vi "IDByteDecoder.vi"(0 "byte1":string="Ò") -> (1 "Type de donnee (ID)":i32, 2 "Ordre/ /(info)":bool, 3 "marche normale/ /(debug)":bool)   [LabVIEW 2010]
doc: "Décodage d'un octet de type de données"
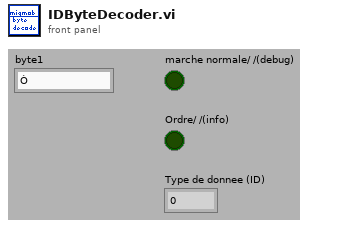
[diagram p1: front panel]
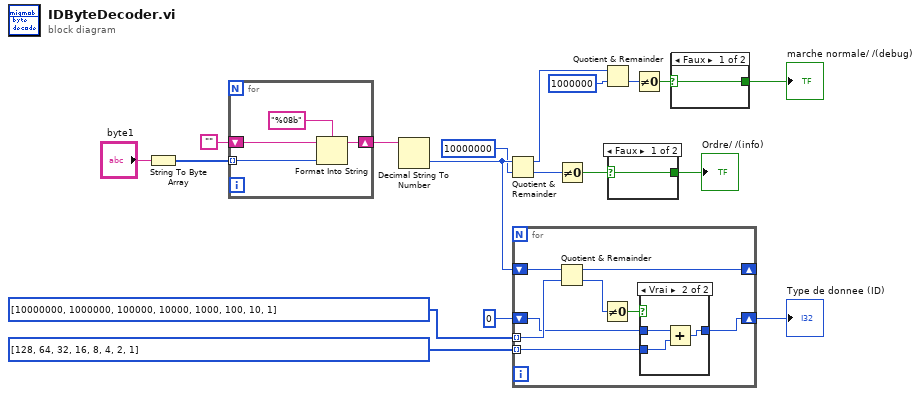
[diagram p0: block diagram]
diagram:
  n1 = String To Byte Array(string="byte1") -> (unsigned byte array=w5:u8[])
  n2 = for {
    tunnel: w5 -> [w22] mode=indexing
    shift-right: [w20] -> w3
    shift-left: "" -> [w21]
    n3 = Format Into String(format string="%08b" ("chaîne de format"), initial string=w21, w22) -> (resulting string=w20:string)  [unwired: 1 in, 1 out]
  }
  n4 = Decimal String To Number(string=w3) -> (number=w16:i32)  [unwired: 2 in, 1 out]
  n5 = Quotient & Remainder(x=w16, y=10000000) -> (x-y*floor(x/y)=w9:i32, floor(x/y)=w7:i32)
  n6 = for {
    tunnel: i32[] [10000000, 1000000, 100000, 10000, 1000, 100, 10, 1] -> [w29] mode=indexing
    shift-right: [w25] -> _
    shift-left: w16 -> [w30]
    shift-right: [w23] -> w18
    shift-left: 0 -> [w26]
    tunnel: i32[] [128, 64, 32, 16, 8, 4, 2, 1] -> [w24] mode=indexing
    n7 = Quotient & Remainder(x=w30, y=w29) -> (x-y*floor(x/y)=w25:i32, floor(x/y)=w28:i32)
    n8 = Not Equal To 0?(x=w28) -> (x != 0?=w27:bool)
    n9 = case shown="Vrai" w27 {
      tunnel: w26 -> [w31 w34]
      tunnel: [w31 w32] -> w23
      tunnel: w24 -> [_ w33]
      frame False {
      }
      frame True {
        n10 = Add(x=w34, y=w33) -> (x+y=w32:i32)
      }
    }
  }
  "Type de donnee (ID)" <- w18
  n11 = Not Equal To 0?(x=w7) -> (x != 0?=w8:bool)
  n12 = Quotient & Remainder(x=w9, y=1000000) -> (floor(x/y)=w13:i32)  [unwired: 1 out]
  n13 = case shown="Faux" w8 {
    selector: w8 -> [w35 w36]
    tunnel: [w35 w36] -> w1
    frame False {
    }
    frame True {
    }
  }
  "Ordre/ /(info)" <- w1
  n14 = Not Equal To 0?(x=w13) -> (x != 0?=w11:bool)
  n15 = case shown="Faux" w11 {
    selector: w11 -> [w37 w38]
    tunnel: [w37 w38] -> w12
    frame False {
    }
    frame True {
    }
  }
  "marche normale/ /(debug)" <- w12
